vi "get_name.vi"(8 "error in (no error)":errorcluster, 11 "GenericPlugin in":refnum<class "GenericComponent.lvclass">) -> (0 "error out":errorcluster, 2 "component name":string, 3 "GenericPlugin out":refnum<class "GenericComponent.lvclass">)   [LabVIEW 2010, in "GenericComponent.lvclass"]
uses:
  GenericComponent.lvclass
  <vilib>/regexp/Match Regular Expression.xnode
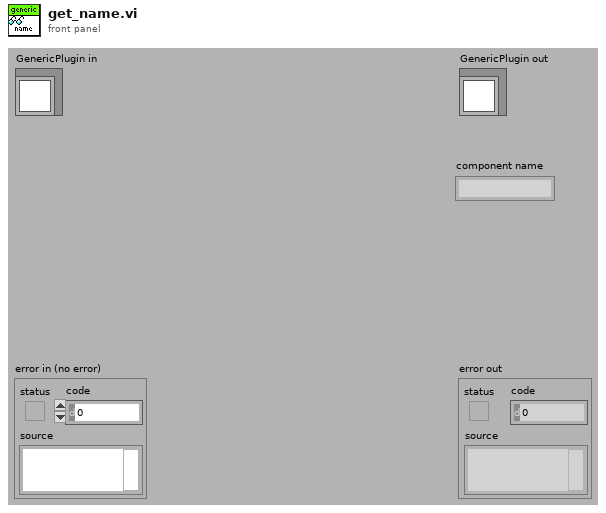
[diagram p1: front panel]
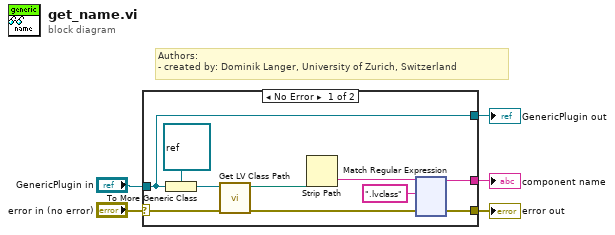
[diagram p0: block diagram]
diagram:
  # "Authors: \n- created by: Dominik Langer, University of Zurich, Switzerland"
  n1 = case shown="No Error" "error in (no error)" {
    selector: "error in (no error)" -> [w11 w128]
    tunnel: [w13 w128] -> w4
    tunnel: [w6 w127] -> w2
    tunnel: "GenericPlugin in" -> [w6 w127]
    tunnel: [w12 _] -> w1
    frame No Error {
      n2 = To More Generic Class(target class=refnum<class> refnum ("LabVIEW Object"), reference=w6) -> (generic class reference=w7:refnum<class>)
      n3 = call <vilib>:"Get LV Class Path.vi"("error in (no error)"=w11, "object"=w7) -> ("error out"=w8:errorcluster, "class path"=w9:path)  [unwired: 8 in]
      n4 = Strip Path(path=w9) -> (name=w15:string)  [unwired: 1 out]
      n5 = xnode "Match Regular Expression"("input string"=w15, "regular expression"=".lvclass", "error in"=w8) -> ("before match"=w12:string, "error out"=w13:errorcluster)  [unwired: 3 in, 3 out]
    }
    frame Error {
    }
  }
  "error out" <- w4
  "GenericPlugin out" <- w2
  "component name" <- w1
